vi "Create Lock.vi"(8 "error in (no error)":errorcluster, 10 "initial lock status (T)":bool=TRUE, 11 "Pointer in":refnum<class "Pointer.lvclass">) -> (0 "error out":errorcluster, 3 "Pointer out":refnum<class "Pointer.lvclass">)   [LabVIEW 2017, in "Memory Manager.lvlib" / "Pointer.lvclass"]
uses:
  Pointer.lvclass
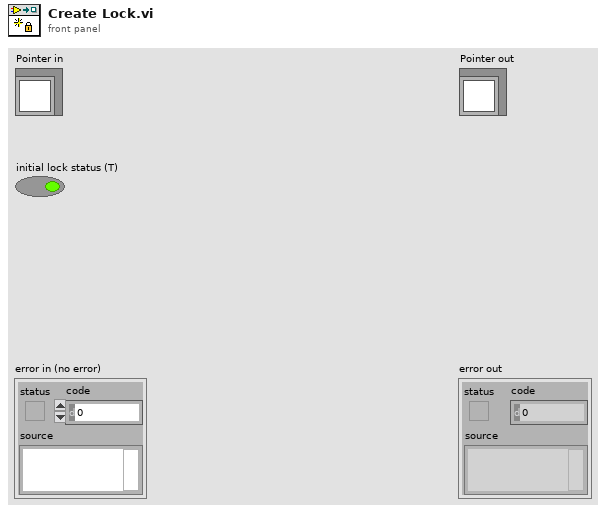
[diagram p1: front panel]
types:
  T1 = cluster{"read mode":enum16{"polling", "blocking"}, "write mode":enum16{"polling", "blocking"}}
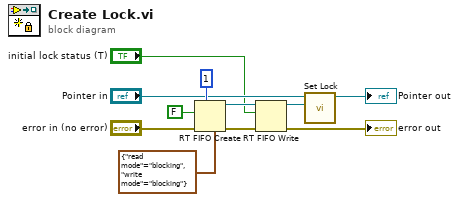
[diagram p0: block diagram]
diagram:
  n1 = RT FIFO Create(1:FALSE, 3:"error in (no error)", 4:u32 1 ("size (10)"), 7:T1 {"read mode"=enum."blocking", "write mode"=enum."blocking"} ("r/w modes (polling,polling)")) -> (8:w8:refnum<k33>, 11:w7:errorcluster)  [unwired: 4 in, 1 out]
  n2 = RT FIFO Write(0:w8, 1:"initial lock status (T)", 3:w7) -> (8:w6:refnum<k33>, 11:→"error out":errorcluster)  [unwired: 2 in, 2 out]
  n3 = call "Set Lock.vi"("lock"=w6, "Pointer in"="Pointer in") -> ("Pointer out"=→"Pointer out":refnum<class "Pointer.lvclass">)  [unwired: 9 in]
